vi "Read.vi"(11 "AppStartupValue in":refnum<class "AppStartupValue.lvclass">) -> (2 "error out":errorcluster, 3 "Events":T1[](array[typedef]))   [LabVIEW 2020, in "Volatus.lvlib" / "AppStartupValue.lvclass"]
uses:
  AppStartupValue.lvclass
  AppStartupValue.lvclass/AppStartupValue.ctl
  Event Level.ctl
  Volatus.lvlib
  Event.ctl
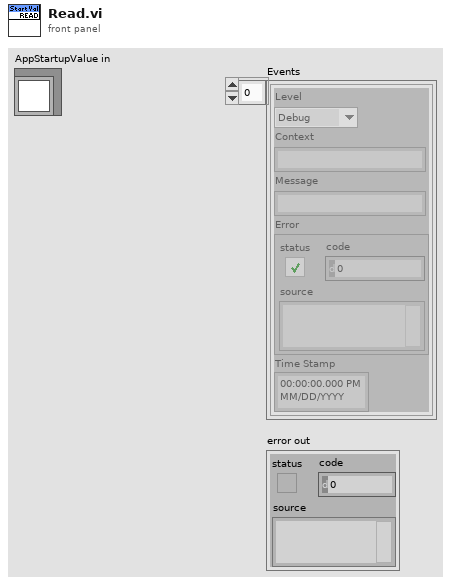
[diagram p1: front panel]
types:
  T1 = typedef "Volatus.lvlib/Event.ctl" = cluster{"Level":T2, "Context":string, "Message":string, "Error":errorcluster, "Time Stamp":timestamp}
  T2 = typedef "Volatus.lvlib/Event Level.ctl" = enum16{"Debug", "Info", "Warning", "Error"}
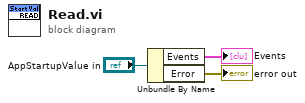
[diagram p0: block diagram]
diagram:
  n1 = Unbundle By Name("AppStartupValue in") -> ("Events"=→"Events":T1[], "Error"=→"error out":errorcluster)
